vi "Format.vi"(0 "VISA IN":refnum<visa-resource-name>, 1 "Measurement Name":string="CH1_S11_1", 2 "Format":string(combo)="MLINear", 5 "error in":errorcluster, 7 "Channel":i32=1) -> (14 "VISA Out":refnum<visa-resource-name>, 19 "error out":errorcluster)   [LabVIEW 2018, in "PNA-X.lvlib"]
uses:
  PNA-X.lvlib
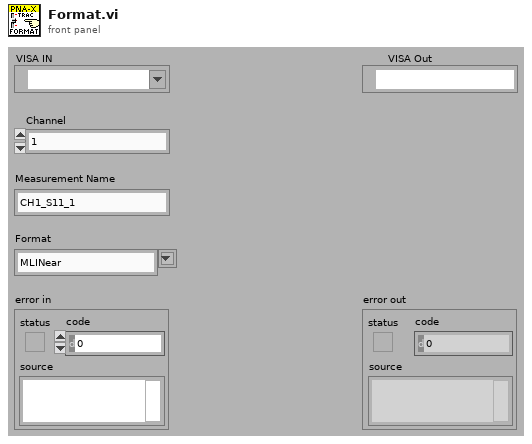
[diagram p1: front panel]
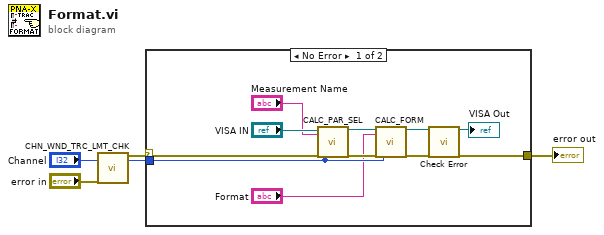
[diagram p0: block diagram]
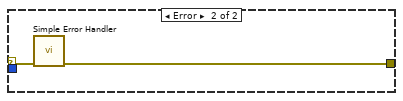
[diagram p2: hidden frame]
diagram:
  n1 = call "CHN_WND_TRC_LMT_CHK.vi"("Channel"="Channel", "error in"="error in") -> ("error out"=w2:errorcluster, "Channel"=w1:i32)  [unwired: 13 in, 3 out]
  n2 = case shown="No Error" w2 {
    selector: w2 -> [w14 w18]
    tunnel: [w16 w17] -> w4
    tunnel: w1 -> [w8 _]
    frame No Error {
      n3 = call "CALC_PAR_SEL.vi"("VISA IN"="VISA IN", "Measurement"="Measurement Name", "error in"=w14, "Channel"=w8) -> ("VISA Out"=w12:refnum<visa-resource-name>, "error out"=w10:errorcluster)  [unwired: 14 in]
      n4 = call "CALC_FORM.vi"("VISA IN"=w12, "Format"="Format", "error in"=w10, "Channel"=w8) -> ("VISA Out"=w11:refnum<visa-resource-name>, "error out"=w9:errorcluster)  [unwired: 14 in]
      n5 = call "Check Error.vi"("VISA Resource Name"=w11, "error in (no error)"=w9) -> ("dup VISA session"=→"VISA Out":refnum<visa-resource-name>, "error out"=w16:errorcluster)  [unwired: 16 in]
    }
    frame Error {
      n6 = call <vilib>:"Simple Error Handler.vi"("error in (no error)"=w18) -> ("error out"=w17:errorcluster)  [unwired: 4 in, 4 out]
    }
  }
  "error out" <- w4
